vi "LV SciSDK INIT FFT.vi"(0 "FFT Name":string, 1 "Acq mode":string(combo)="blocking", 5 "Decimator":u32, 7 "Timeout":i32=5000, 9 "Handle In":T2, 11 "error in (no error)":errorcluster) -> (10 "FFT Handle Out":T1, 15 "error out":errorcluster)   [LabVIEW 2021]
uses:
  SciSDK_Labview.lvlib
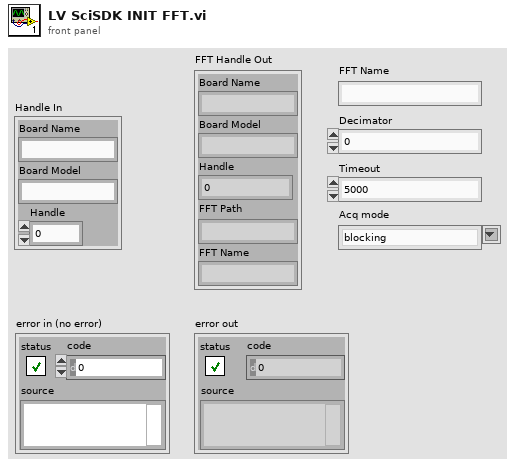
[diagram p1: front panel]
types:
  T1 = cluster{"Board Name":string, "Board Model":string, "Handle":u64, "FFT Path":string, "FFT Name":string}
  T2 = cluster{"Board Name":string, "Board Model":string, "Handle":u64}
  T3 = cluster{"Board Name":string, "Board Model":string, "Handle":u64, string, "FFT Name":string}
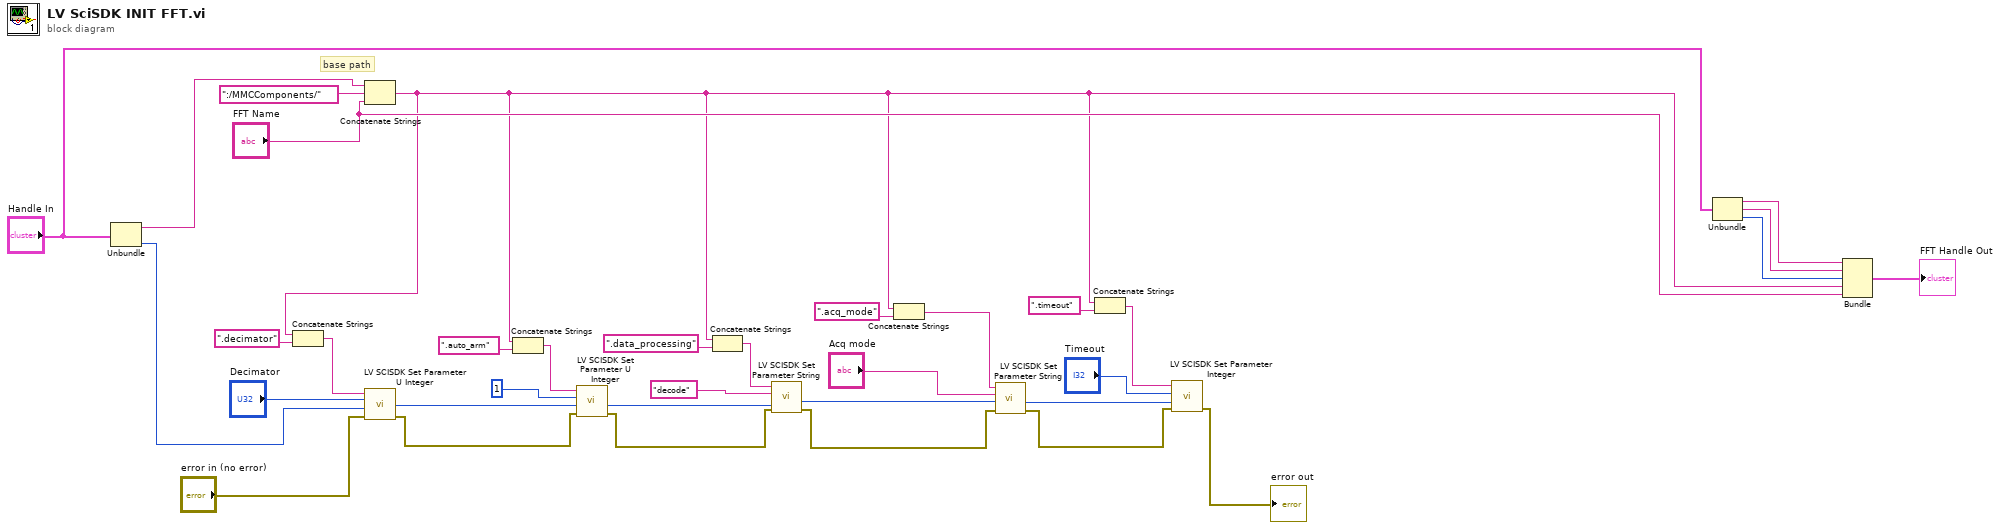
[diagram p0: block diagram]
diagram:
  # "base path"
  n1 = Unbundle("Handle In") -> ("Board Name"=w34:string, "Handle"=w21:u64)  [unwired: 1 out]
  n2 = Concatenate Strings(w34, ":/MMCComponents/" ("string"), "FFT Name") -> (w1:string)
  n3 = Concatenate Strings(w1, ".decimator" ("string")) -> (w20:string)
  n4 = call "LV SCISDK Set Parameter U Integer.vi"("error in (no error)"="error in (no error)", "handle"=w21, "value"="Decimator", "Path"=w20) -> ("error out"=w16:errorcluster, "handle out"=w17:u64)  [unwired: 5 in, 1 out]
  n5 = Concatenate Strings(w1, ".auto_arm" ("string")) -> (w18:string)
  n6 = call "LV SCISDK Set Parameter U Integer.vi"("error in (no error)"=w16, "handle"=w17, "value"=u32 1, "Path"=w18) -> ("error out"=w14:errorcluster, "handle out"=w15:u64)  [unwired: 5 in, 1 out]
  n7 = Concatenate Strings(w1, ".data_processing" ("string")) -> (w12:string)
  n8 = call "LV SCISDK Set Parameter String.vi"("error in (no error)"=w14, "handle"=w15, "value"="decode", "Path"=w12) -> ("error out"=w11:errorcluster, "handle out"=w10:u64)  [unwired: 5 in, 1 out]
  n9 = Concatenate Strings(w1, ".acq_mode" ("string")) -> (w8:string)
  n10 = call "LV SCISDK Set Parameter String.vi"("error in (no error)"=w11, "handle"=w10, "value"="Acq mode", "Path"=w8) -> ("error out"=w3:errorcluster, "handle out"=w4:u64)  [unwired: 5 in, 1 out]
  n11 = Concatenate Strings(w1, ".timeout" ("string")) -> (w6:string)
  n12 = call "LV SCISDK Set Parameter Integer.vi"("error in (no error)"=w3, "handle"=w4, "value"="Timeout", "Path"=w6) -> ("error out"=→"error out":errorcluster)  [unwired: 5 in, 2 out]
  n13 = Unbundle("Handle In") -> ("Board Name"=w33:string, "Board Model"=w32:string, "Handle"=w31:u64)
  n14 = Bundle("Board Name"=w33, "Board Model"=w32, "Handle"=w31, w1, "FFT Name"="FFT Name") -> (→"FFT Handle Out":T3)  [unwired: 1 in]
